vi "(4-20) mA to Lh.vi"(8 "x":dbl, 11 "flowMax":dbl) -> (3 "flowOut":dbl)   [LabVIEW 2021]
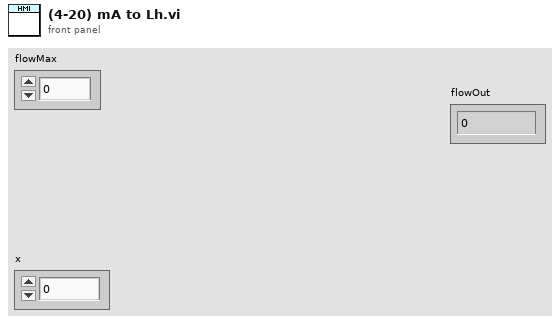
[diagram p1: front panel]
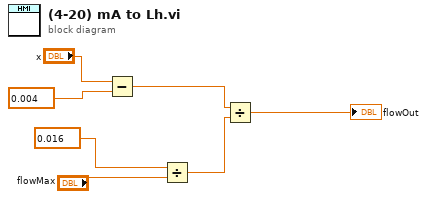
[diagram p0: block diagram]
diagram:
  n1 = Subtract(x="x", y=0.004) -> (x-y=w1:dbl)
  n2 = Divide(x=0.016 ("Amax"), y="flowMax") -> (x/y=w5:dbl)
  n3 = Divide(x=w1, y=w5) -> (x/y=→"flowOut":dbl)
